vi "Initialize From Settings.vi"(8 "error in (no error)":errorcluster, 9 "settings version":T1, 10 "settings":cluster{"key":string, "value":string}[](array[cluster]), 11 "UDP Tx Transfer Configuration in":refnum<class "UDP Transfer Tx Configuration.lvclass">) -> (0 "error out":errorcluster, 3 "UDP Tx Transfer Configuration out":refnum<class "UDP Transfer Tx Configuration.lvclass">)   [LabVIEW 2017, in "UDP Transfer Tx Configuration.lvclass"]
uses:
  UDP Transfer Tx Configuration.lvclass
  Typedefs/DSF Version Info.ctl
  UDP Transfer Tx Configuration.lvclass/UDP Transfer Tx Configuration.ctl
  DSF Core.lvlib
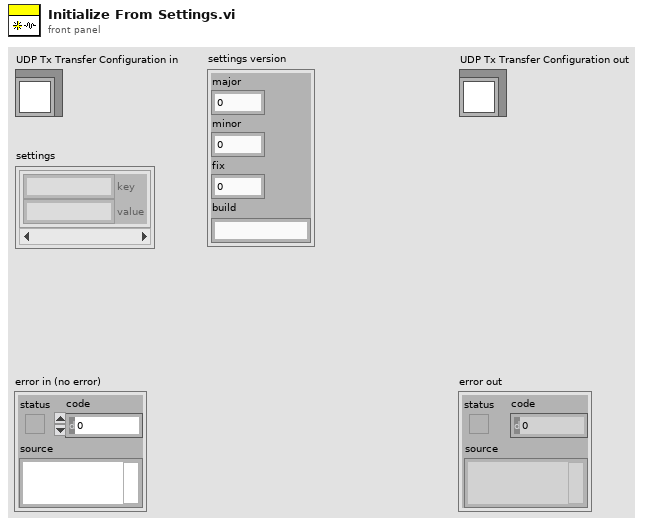
[diagram p1: front panel]
types:
  T1 = typedef "DSF Core.lvlib/DSF Version Info.ctl" = cluster{"major":u32, "minor":u32, "fix":u32, "build":string}
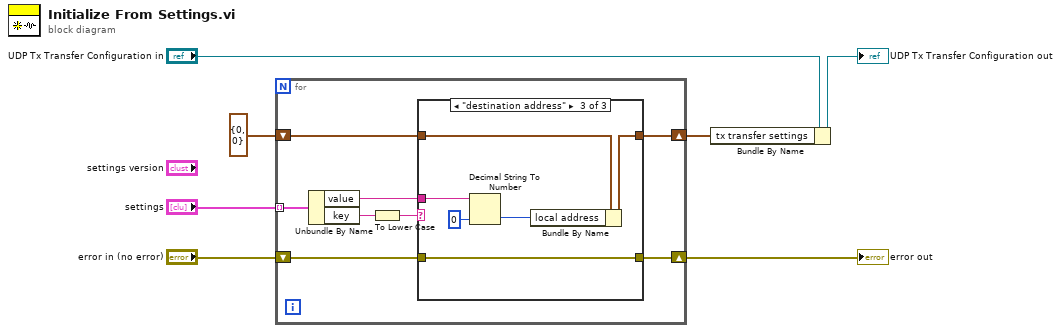
[diagram p0: block diagram]
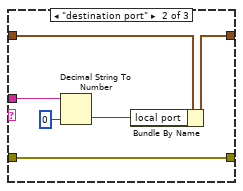
[diagram p3: hidden frame]
diagram:
  n1 = for {
    shift-right: [w8] -> w5
    shift-left: "error in (no error)" -> [w14]
    shift-right: [w10] -> w2
    shift-left: cluster{"local port":u16, "local address":u32} {"local port"=0, "local address"=0} ("thread settings") -> [w11]
    tunnel: "settings" -> [w15] mode=indexing
    n2 = Unbundle By Name(w15) -> ("value"=w12:string, "key"=w13:string)
    n3 = To Lower Case(string=w13) -> (all lower case string=w9:string)
    n4 = case shown="\"destination address\"" w9 {
      tunnel: w14 -> [w16 w21 w27]
      tunnel: w12 -> [_ w20 w25]
      tunnel: w11 -> [w17 w23 w29]
      tunnel: [w17 w22 w28] -> w10
      tunnel: [w16 w21 w27] -> w8
      frame Default {
        # "Unknown Setting."
      }
      frame "destination port" {
        n5 = Decimal String To Number(string=w20, default (0L)=u16 0 ("default (0 I32)")) -> (number=w19:u16)  [unwired: 1 in, 1 out]
        n6 = Bundle By Name(cluster=w23, "local port"=w19) -> (w22:cluster{"local port":u16, "local address":u32})
      }
      frame "destination address" {
        n7 = Decimal String To Number(string=w25, default (0L)=u32 0 ("default (0 I32)")) -> (number=w24:u32)  [unwired: 1 in, 1 out]
        n8 = Bundle By Name(cluster=w29, "local address"=w24) -> (w28:cluster{"local port":u16, "local address":u32})
      }
    }
  }
  "error out" <- w5
  n9 = Bundle By Name(cluster="UDP Tx Transfer Configuration in", "tx transfer settings"=w2) -> (→"UDP Tx Transfer Configuration out":refnum<class "UDP Transfer Tx Configuration.lvclass">)
